vi "Create Hook.vi"() -> ()   [LabVIEW 2018, in "Tools Menu.lvlib"]
uses:
  Tools Menu.lvlib
  Toolkit/Support/Post-Bury Template.vi
  Toolkit/Support/Pre-Dig Template.vi
  Toolkit/Support/Post-Dig Template.vi
  Toolkit/Support/Pre-Reanimate Template.vi
  Toolkit/Support/Post-Reanimate Template.vi
  Toolkit/Support/Pre-Smite Template.vi
  Toolkit/Support/Post-Smite Template.vi
  Toolkit/Toolkit.lvlib
panel:
  in  "Cancel":bool
  in  "Create":bool
  in  "Execution":T1(ring)
  in  "Destination":path
  in  "For":T2(ring)=enum."User"
  in  "When":enum16{"Pre (Before)", "Post (After)"}(ring)
  in  "Action":enum16{"Bury", "Dig", "Reanimate", "Smite"}(ring)
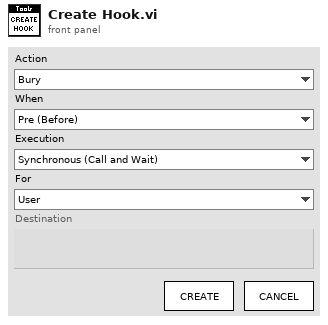
[diagram p1: front panel]
types:
  T1 = enum16{"Synchronous (Call and Wait)", "Asynchronous (Call and Forget)"}
  T2 = enum16{"System", "User", "Project (Visible)", "Project (Hidden)", "Custom..."}
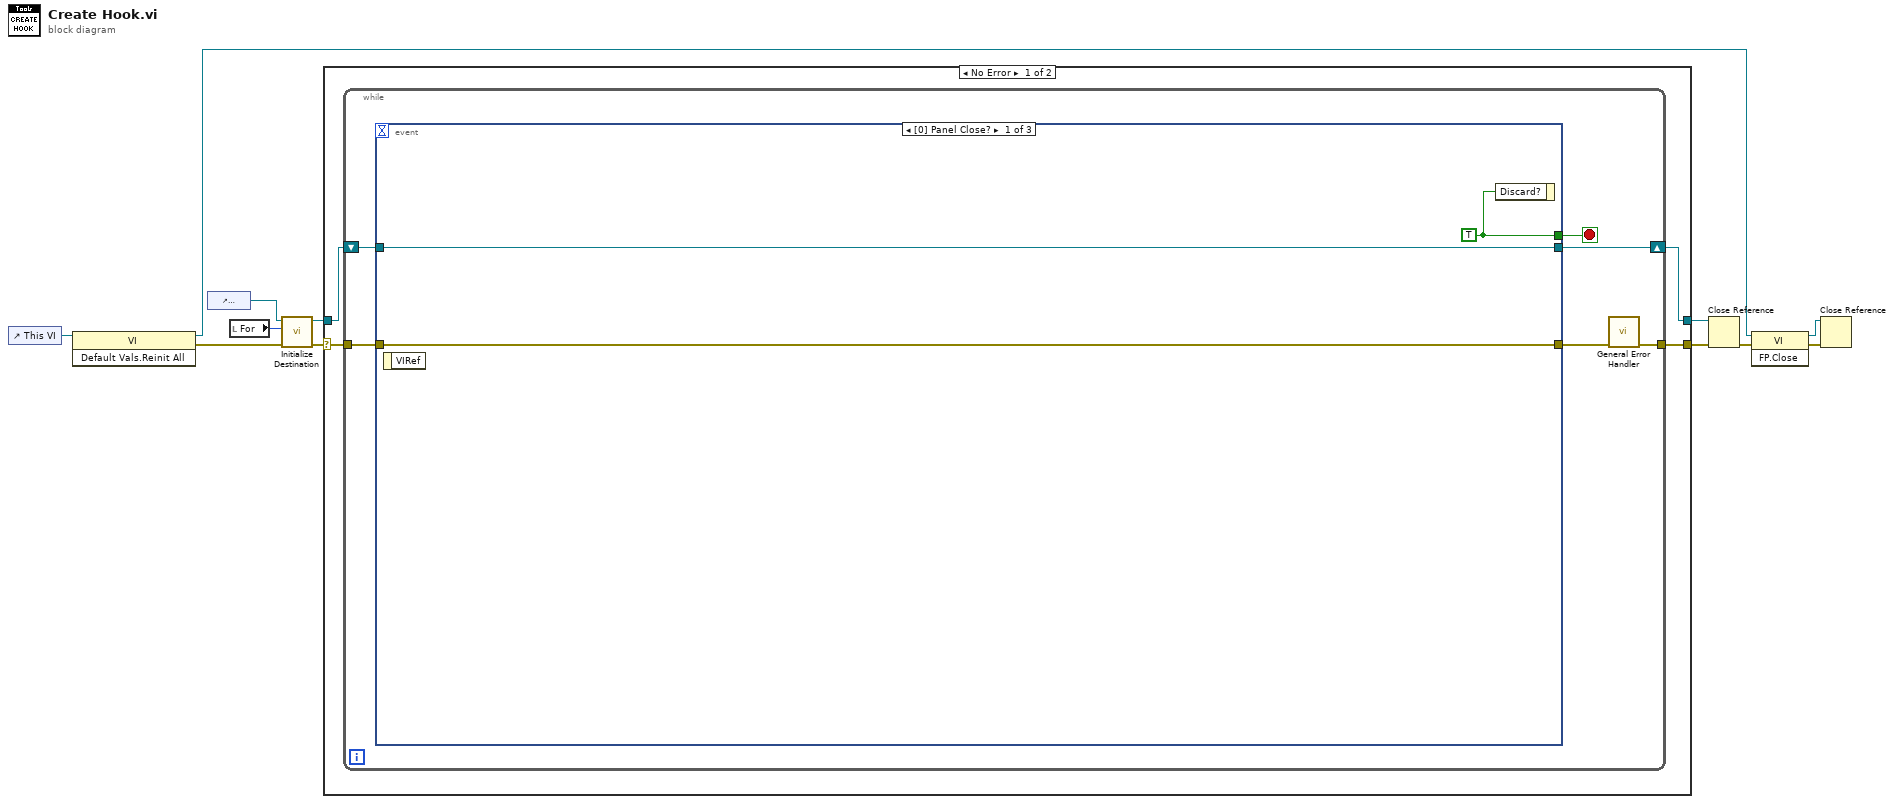
[diagram p0: block diagram]
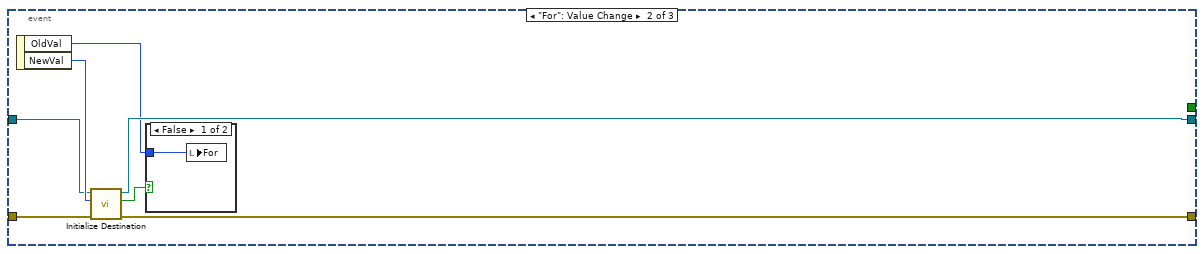
[diagram p2: hidden frame]
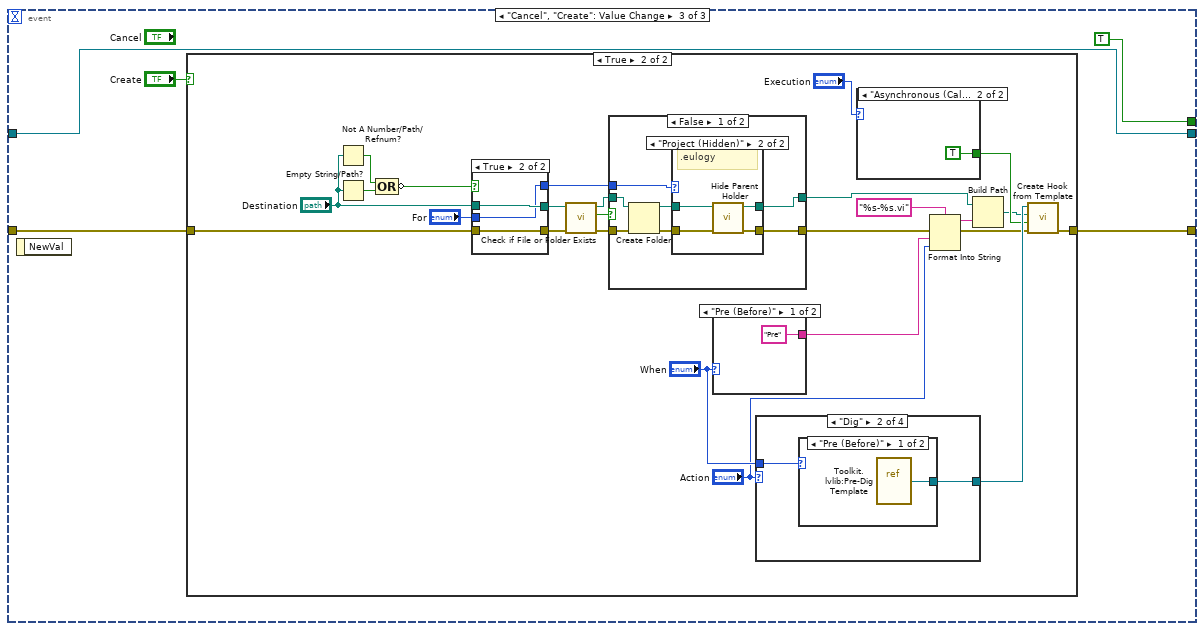
[diagram p4: hidden frame]
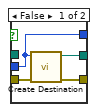
[diagram p6: hidden frame]
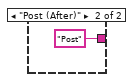
[diagram p9: hidden frame]
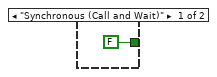
[diagram p10: hidden frame]
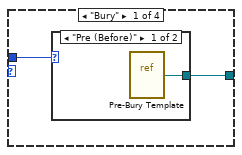
[diagram p11: hidden frame]
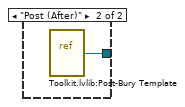
[diagram p12: hidden frame]
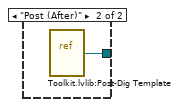
[diagram p13: hidden frame]
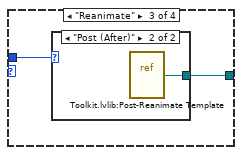
[diagram p14: hidden frame]
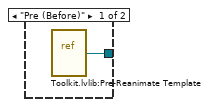
[diagram p15: hidden frame]
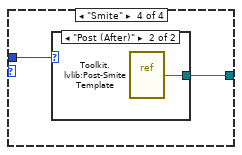
[diagram p16: hidden frame]
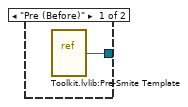
[diagram p17: hidden frame]
diagram:
  n1 = control-ref of="This VI"() -> (w12:refnum<vi>)
  n2 = invoke class="VI" method="Default Vals.Reinit All"(reference=w12) -> (reference out=w1:refnum<vi>, error out=w5:errorcluster)  [unwired: 2 in, 1 out]
  n3 = control-ref of="Destination"() -> (w11:refnum<vi>)
  n4 = local read "For"() -> (w9:T2)
  n5 = call "Initialize Destination.vi"("Error In"=w5, "For"=w9, "Destination In"=w11) -> ("Error Out"=w6:errorcluster, "Destination Out"=w10:refnum<vi>)  [unwired: 6 in, 1 out]
  n6 = case shown="No Error" w6 {
    selector: w6 -> [w13 w107]
    tunnel: w10 -> [w16 w108]
    tunnel: [w15 w108] -> w8
    tunnel: [w14 w107] -> w7
    frame No Error {
      n7 = while {
        tunnel: w13 -> [w19]
        shift-right: [w18] -> w15
        shift-left: w16 -> [w20]
        tunnel: [w17] -> w14
        stop <- w22 stop-if-true
        n8 = event shown="[0] Panel Close?" {
          selector: _ -> [_ _ _]
          dyn-events: _ -> [_ _ _]
          timeout: _ -> [_ _ _]
          tunnel: [w23 _ TRUE] -> w22
          tunnel: [w24 w32 w36] -> w21
          tunnel: w20 -> [w25 w30 w35]
          tunnel: w19 -> [w24 w29 w34]
          tunnel: [w25 w28 w35] -> w18
          event Panel Close? {
            w23 = TRUE
            n9 = event-data() -> ()  [unwired: 1 in, 1 out]
            n10 = event-data("Discard?"=w23) -> ()  [unwired: 1 in, 1 out]
          }
          event "For": Value Change {
            n11 = event-data() -> ("OldVal"=w26:T2, "NewVal"=w31:T2)  [unwired: 1 in]
            n12 = call "Initialize Destination.vi"("Error In"=w29, "For"=w31, "Destination In"=w30) -> ("Error Out"=w32:errorcluster, "Change Made?"=w27:bool, "Destination Out"=w28:refnum<vi>)  [unwired: 6 in]
            n13 = case shown="False" w27 {
              tunnel: w26 -> [w33 _]
              frame False {
                n14 = local write "For"(w33) -> ()
              }
              frame True {
              }
            }
          }
          event "Cancel", "Create": Value Change {
            n15 = event-data() -> ()  [unwired: 1 in, 1 out]
            n16 = case shown="True" "Create" {
              tunnel: [w39 w61] -> w36
              tunnel: w34 -> [w39 w42]
              frame False {
              }
              frame True {
                n17 = Not A Number/Path/Refnum?(number/path/refnum="Destination") -> (NaN/Path/Refnum?=w47:bool)
                n18 = Empty String/Path?(string/path="Destination") -> (empty?=w48:bool)
                n19 = Compound Arithmetic op=OR(w47, w48) -> (invert w46:bool)
                n20 = case shown="True" w46 {
                  tunnel: "Destination" -> [_ w71]
                  tunnel: [w67 w71] -> w44
                  tunnel: [w68 w70] -> w43
                  tunnel: w42 -> [w66 w70]
                  tunnel: "For" -> [w65 w69]
                  tunnel: [w65 w69] -> w40
                  frame False {
                    n21 = call "Create Destination.vi"("Error In"=w66, "For"=w65) -> ("Error Out"=w68:errorcluster, "Destination"=w67:path)  [unwired: 8 in]
                  }
                  frame True {
                  }
                }
                n22 = call <vilib>:"Check if File or Folder Exists.vi"("error in (no error)"=w43, "path"=w44) -> ("error out"=w52:errorcluster, "file or folder exists?"=w54:bool, "dup path"=w53:path)  [unwired: 7 in]
                n23 = case shown="False" w54 {
                  tunnel: w53 -> [w78 w86]
                  tunnel: w52 -> [w77 w85]
                  tunnel: [w72 w86] -> w51
                  tunnel: [w74 w85] -> w49
                  tunnel: w40 -> [w76 _]
                  frame False {
                    n24 = Create Folder(path (use dialog)=w78, error in=w77) -> (created path=w73:path, error out=w75:errorcluster)  [unwired: 1 in, 1 out]
                    n25 = case shown="\"Project (Hidden)\"" w76 {
                      tunnel: w75 -> [w79 w84]
                      tunnel: [w79 w83] -> w74
                      tunnel: w73 -> [w80 w82]
                      tunnel: [w80 w81] -> w72
                      frame "System", Default {
                      }
                      frame "Project (Hidden)" {
                        # ".eulogy"
                        n26 = call "Hide Parent Holder.vi"("Error In"=w84, "Child Folder In"=w82) -> ("Error Out"=w83:errorcluster, "Child Folder Out"=w81:path)  [unwired: 8 in]
                      }
                    }
                  }
                  frame True {
                  }
                }
                n27 = case shown="\"Pre (Before)\"" "When" {
                  tunnel: ["Pre" "Post"] -> w60
                  frame "Pre (Before)" {
                  }
                  frame "Post (After)" {
                  }
                }
                n28 = case shown="\"Dig\"" "Action" {
                  tunnel: "When" -> [w92 w96 w100 w104]
                  tunnel: [w91 w95 w99 w103] -> w64
                  frame "Bury" {
                    n29 = case shown="\"Pre (Before)\"" w92 {
                      tunnel: [w93 w94] -> w91
                      frame "Pre (Before)" {
                        n30 = vi-ref "Pre-Bury Template.vi"() -> (w93:refnum<vi>)
                      }
                      frame "Post (After)" {
                        n31 = vi-ref "Toolkit.lvlib:Post-Bury Template.vi"() -> (w94:refnum<vi>)
                      }
                    }
                  }
                  frame "Dig" {
                    n32 = case shown="\"Pre (Before)\"" w96 {
                      tunnel: [w97 w98] -> w95
                      frame "Pre (Before)" {
                        n33 = vi-ref "Toolkit.lvlib:Pre-Dig Template.vi"() -> (w97:refnum<vi>)
                      }
                      frame "Post (After)" {
                        n34 = vi-ref "Toolkit.lvlib:Post-Dig Template.vi"() -> (w98:refnum<vi>)
                      }
                    }
                  }
                  frame "Reanimate" {
                    n35 = case shown="\"Post (After)\"" w100 {
                      tunnel: [w101 w102] -> w99
                      frame "Pre (Before)" {
                        n36 = vi-ref "Toolkit.lvlib:Pre-Reanimate Template.vi"() -> (w101:refnum<vi>)
                      }
                      frame "Post (After)" {
                        n37 = vi-ref "Toolkit.lvlib:Post-Reanimate Template.vi"() -> (w102:refnum<vi>)
                      }
                    }
                  }
                  frame "Smite" {
                    n38 = case shown="\"Post (After)\"" w104 {
                      tunnel: [w105 w106] -> w103
                      frame "Pre (Before)" {
                        n39 = vi-ref "Toolkit.lvlib:Pre-Smite Template.vi"() -> (w105:refnum<vi>)
                      }
                      frame "Post (After)" {
                        n40 = vi-ref "Toolkit.lvlib:Post-Smite Template.vi"() -> (w106:refnum<vi>)
                      }
                    }
                  }
                }
                n41 = case shown="\"Asynchronous (Call and Forget)\"" "Execution" {
                  tunnel: [FALSE TRUE] -> w62
                  frame "Synchronous (Call and Wait)" {
                  }
                  frame "Asynchronous (Call and Forget)" {
                  }
                }
                n42 = Format Into String(format string="%s-%s.vi", error in=w49, w60, "Action") -> (resulting string=w55:string, error out=w56:errorcluster)  [unwired: 1 in]
                n43 = Build Path(base path=w51, name or relative path=w55) -> (appended path=w50:path)
                n44 = call "Create Hook from Template.vi"("Error In"=w56, "Call and Forget?"=w62, "Save Destination"=w50, "VI Template"=w64) -> ("Error Out"=w61:errorcluster)  [unwired: 7 in]
              }
            }
          }
        }
        n45 = call <vilib>:"General Error Handler.vi"("error in (no error)"=w21) -> ("error out"=w17:errorcluster)  [unwired: 10 in, 4 out]
      }
    }
    frame Error {
    }
  }
  n46 = Close Reference(reference=w8, error in (no error)=w7) -> (error out=w4:errorcluster)
  n47 = invoke class="VI" method="FP.Close"(reference=w1, error in=w4) -> (reference out=w2:refnum<vi>, error out=w3:errorcluster)  [unwired: 1 in, 1 out]
  n48 = Close Reference(reference=w2, error in (no error)=w3) -> ()  [unwired: 1 out]
